vi "track2behavior.vi"(7 "ParallelPoolID":i32, 8 "error in (no error)":errorcluster, 10 "Track In":T2={"Track Centroid Positions (Camera Pixel)"=[], "Within Track Index"=0, "Camera Buffer Indecies"=[], "Area (Camera Pixels)"=0, "Speed (mm/s)"=0.0, "Direction (radians)"=0.0, "Centerline Positions (Camera Pixel)"=[], "Ellipse Ratio"=0.0, "Termination Reason"=enum."StillActive", "Track Index"=0, "Bounding Rect Left"=0, "Bounding Rect Top"=0, "Bounding Rect Right"=0, "Bounding Rect Bottom"=0, "Mature Camera Buffer"=-1, "Start Camera Buffer Index"=0, "Reverse Started Camera Buffer"=-1}, 11 "Original Worm Image":T1) -> (0 "error out":errorcluster, 2 "Track Out":T2={"Track Centroid Positions (Camera Pixel)"=[], "Within Track Index"=0, "Camera Buffer Indecies"=[], "Area (Camera Pixels)"=0, "Speed (mm/s)"=0.0, "Direction (radians)"=0.0, "Centerline Positions (Camera Pixel)"=[], "Ellipse Ratio"=0.0, "Termination Reason"=enum."StillActive", "Track Index"=0, "Bounding Rect Left"=0, "Bounding Rect Top"=0, "Bounding Rect Right"=0, "Bounding Rect Bottom"=0, "Mature Camera Buffer"=-1, "Start Camera Buffer Index"=0, "Reverse Started Camera Buffer"=-1})   [LabVIEW 2019]
uses:
  WormTrackSnippetCluster.ctl
  TrackTerminationReasonEnum.ctl
  <vilib>/vision/Image Controls.llb/IMAQ Image.ctl
  iterative_thinned_image_to_segment.vi
  pixel_XY_to_1D_index.vi
  thinned_image_to_centerline.vi/a49f2ef7-d53c-4424-bee3-5857753b5dab.vi
  iterative_segments_to_centerline.vi
  1D_index_to_pixel_XY.vi
  interp_1d_nearest.vi
  euclidean_distance_double.vi
  flip_2D_single_array_td.vi
  linspace_double.vi
  iterative_segments_to_centerline_oneiteration.vi
  DebugGlobal.vi
  ParametersGlobal.vi
  <vilib>/gmath/interp.llb/Search Ordered Table.vi
  <vilib>/vision/NI_Vision_Development_Module.lvlib
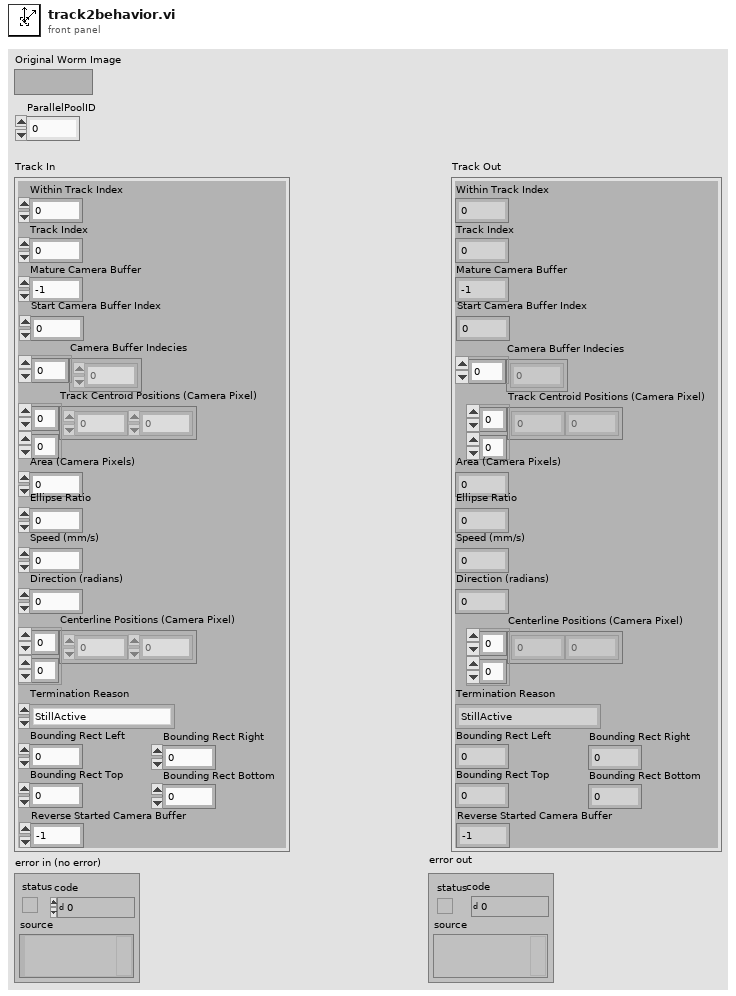
[diagram p1: front panel]
types:
  T1 = typedef "IMAQ Image.ctl" = refnum<image>
  T2 = typedef "WormTrackSnippetCluster.ctl" = cluster{"Track Centroid Positions (Camera Pixel)":sgl[][], "Within Track Index":i32, "Camera Buffer Indecies":i32[], "Area (Camera Pixels)":i32, "Speed (mm/s)":sgl, "Direction (radians)":sgl, "Centerline Positions (Camera Pixel)":sgl[][], "Ellipse Ratio":sgl, "Termination Reason":T3, "Track Index":i32, "Bounding Rect Left":i32, "Bounding Rect Top":i32, "Bounding Rect Right":i32, "Bounding Rect Bottom":i32, "Mature Camera Buffer":i32, "Start Camera Buffer Index":i32, "Reverse Started Camera Buffer":i32}
  T3 = typedef "TrackTerminationReasonEnum.ctl" = enum16{"StillActive", "MaxDisplacement", "NoBlobsLeft", "AreaIncrease", "AreaDecrease", "ExperimentEnded"}
  T4 = typedef "Particle Parameters" = i32
  T5 = cluster{"Left":i32, "Top":i32, "Right":i32, "Bottom":i32}
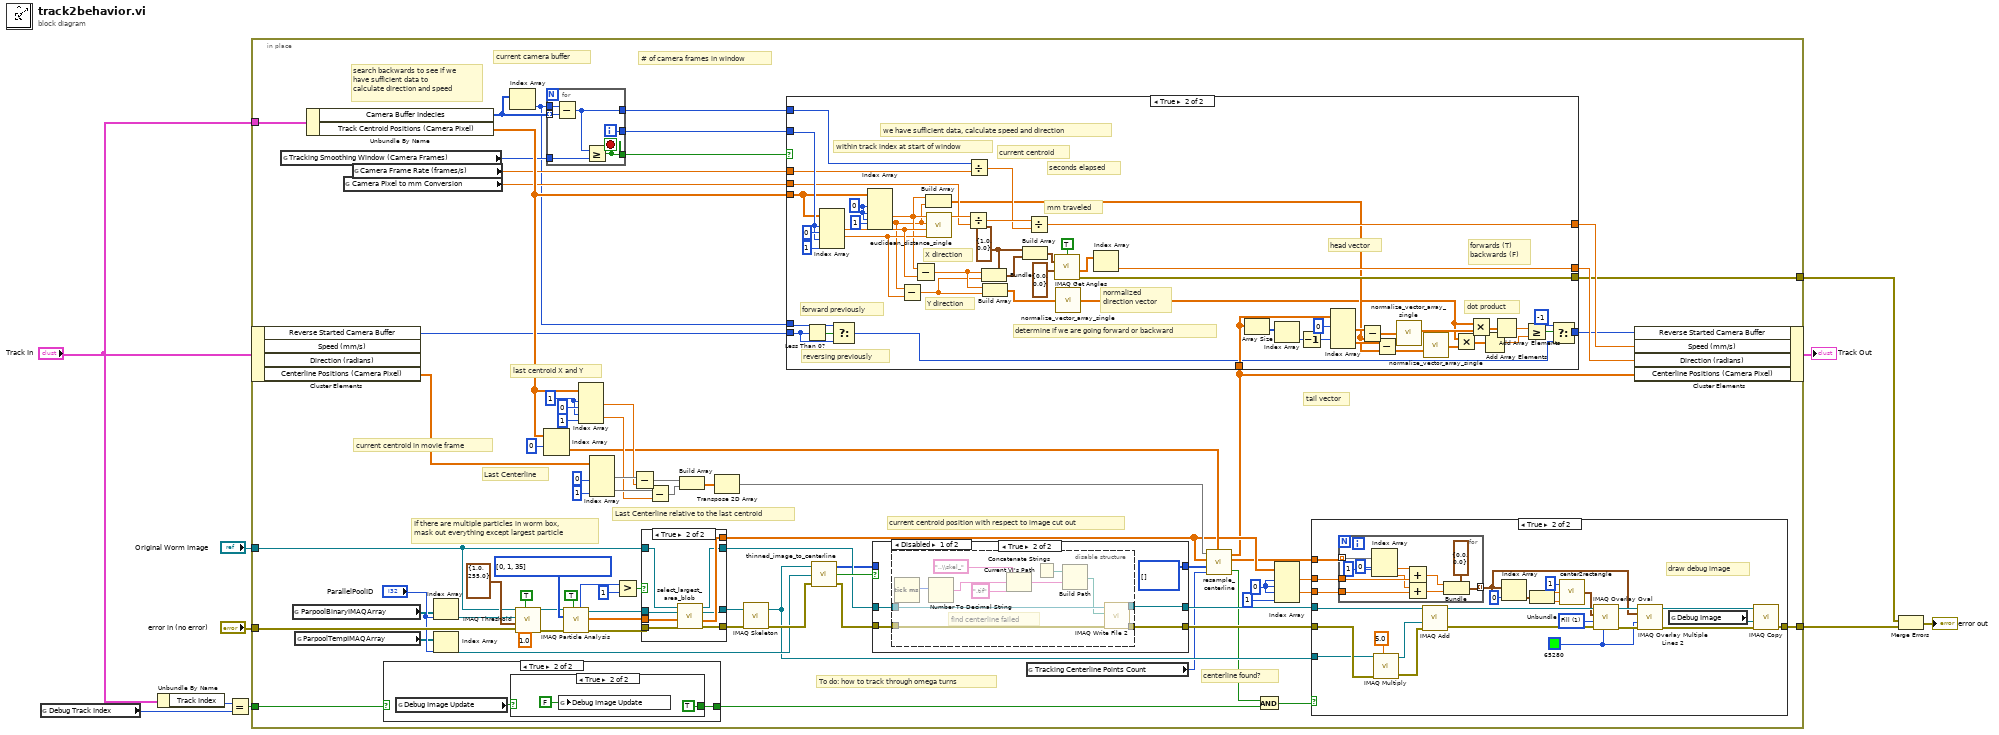
[diagram p0: block diagram]
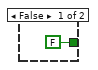
[diagram p2: hidden frame]
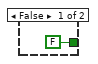
[diagram p3: hidden frame]
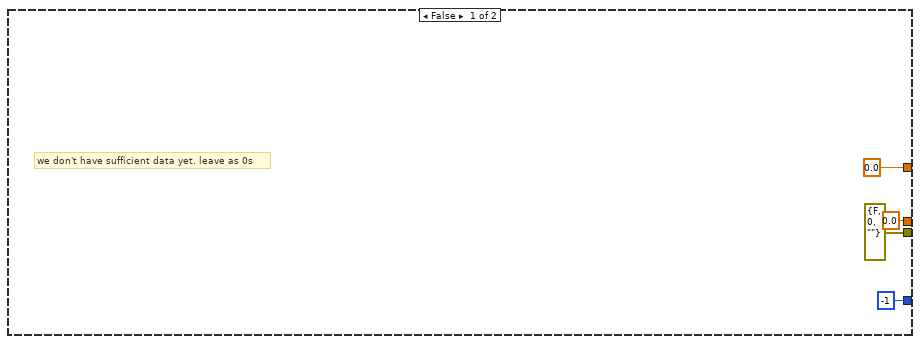
[diagram p8: hidden frame]
diagram:
  n1 = global read "DebugGlobal.vi" "Debug Track Index"() -> (w3:i32)
  n2 = Unbundle By Name("Track In") -> ("Track Index"=w4:i32)
  n3 = Equal?(x=w4, y=w3) -> (x = y?=w2:bool)
  n4 = in-place {
    in-place-border: "Track In" -> [w27]
    in-place-border: "error in (no error)" -> [w79]
    in-place-border: [w25] -> w7
    in-place-border: "Original Worm Image" -> [w65]
    in-place-border: [w66] -> w5
    in-place-border: w2 -> [w12]
    w22 = 1 ("index (row)")
    w36 = 0 ("index (row)")
    w75 = T4[] [0, 1, 35] items=["Center of Mass X", "Center of Mass Y", "First Pixel X", "First Pixel Y", "Bounding Rect Left", "Bounding Rect Top", "Bounding Rect Right", "Bounding Rect Bottom", "Max Feret Diameter Start X", "Max Feret Diameter Start Y", "Max Feret Diameter End X", "Max Feret Diameter End Y", "Max Horiz. Segment Length Left", "Max Horiz. Segment Length Right", "Max Horiz. Segment Length Row", "-", "Bounding Rect Width", "Bounding Rect Height", "Bounding Rect Diagonal", "Perimeter", "Convex Hull Perimeter", "Holes' Perimeter", "Max Feret Diameter", "Equivalent Ellipse Major Axis", "Equivalent Ellipse Minor Axis", "Equivalent Ellipse Minor Axis (Feret)", "Equivalent Rect Long Side", "Equivalent Rect Short Side", "Equivalent Rect Diagonal", "Equivalent Rect Short Side (Feret)", "Average Horiz. Segment Length", "Average Vert. Segment Length", "Hydraulic Radius", "Waddel Disk Diameter", "-", "Area", "Holes' Area", "Particle & Holes' Area", "Convex Hull Area", "Image Area", "-", "Number of Holes", "Number of Horiz. Segments", "Number of Vert. Segments", "-", "Orientation", "Max Feret Diameter Orientation", "-", "% Area/Image Area", "% Area/(Particle & Holes' Area)", "Ratio of Equivalent Ellipse Axes", "Ratio of Equivalent Rect Sides", "-", "Elongation Factor", "Compactness Factor", "Heywood Circularity Factor", "Type Factor", "-", "Sum X", "Sum Y", "Sum XX", "Sum XY", "Sum YY", "Sum XXX", "Sum XXY", "Sum XYY", "Sum YYY", "-", "Moment of Inertia XX", "Moment of Inertia XY", "Moment of Inertia YY", "Moment of Inertia XXX", "Moment of Inertia XXY", "Moment of Inertia XYY", "Moment of Inertia YYY", "Norm. Moment of Inertia XX", "Norm. Moment of Inertia XY", "Norm. Moment of Inertia YY", "Norm. Moment of Inertia XXX", "Norm. Moment of Inertia XXY", "Norm. Moment of Inertia XYY", "Norm. Moment of Inertia YYY", "Hu Moment 1", "Hu Moment 2", "Hu Moment 3", "Hu Moment 4", "Hu Moment 5", "Hu Moment 6", "Hu Moment 7"] ("Pixel Measurements")
    # "current camera buffer"
    # "tail vector"
    # "# of camera frames in window"
    # "If there are multiple particles in worm box, \nmask out everything except largest particle"
    # "centerline found?"
    # "current centroid position with respect to image cut out"
    # "To do: how to track through omega turns"
    # "current centroid in movie frame"
    # "Last Centerline"
    # "last centroid X and Y"
    # "Last Centerline relative to the last centroid"
    # "search backwards to see if we \nhave sufficient data to \ncalculate direction and speed"
    n5 = in-place-cluster #1("Track In") -> ("Reverse Started Camera Buffer"=w18:i32, "Centerline Positions (Camera Pixel)"=w54:sgl[][])  [unwired: 2 out]
    n6 = global read "ParametersGlobal.vi" "Tracking Smoothing Window (Camera Frames)"() -> (w32:i32)
    n7 = global read "ParametersGlobal.vi" "ParpoolBinaryIMAQArray"() -> (w28:T1[])
    n8 = global read "ParametersGlobal.vi" "ParpoolTempIMAQArray"() -> (w29:T1[])
    n9 = Unbundle By Name(w27) -> ("Camera Buffer Indecies"=w84:i32[], "Track Centroid Positions (Camera Pixel)"=w41:sgl[][])
    n10 = global read "ParametersGlobal.vi" "Camera Pixel to mm Conversion"() -> (w30:sgl)
    n11 = global read "ParametersGlobal.vi" "Camera Frame Rate (frames/s)"() -> (w31:sgl)
    n12 = case shown="True" w12 {
      tunnel: [FALSE w87] -> w11
      frame False {
      }
      frame True {
        n13 = global read "DebugGlobal.vi" "Debug Image Update"() -> (w88:bool)
        n14 = case shown="True" w88 {
          tunnel: [FALSE TRUE] -> w87
          frame False {
          }
          frame True {
            n15 = global write "DebugGlobal.vi" "Debug Image Update"(FALSE ("Debug Image Update")) -> ()
          }
        }
      }
    }
    n16 = Index Array(array=w28, index="ParallelPoolID") -> (element=w26:T1)
    n17 = Index Array(array=w29, index="ParallelPoolID") -> (element=w62:T1)
    n18 = Index Array(array=w84) -> (element=w13:i32)  [unwired: 1 in]
    n19 = call "IMAQ Threshold"("Replace Value"=sgl 1.0, "Keep/Replace Value (Replace)"=TRUE, "error in (no error)"=w79, "Range"=cluster{"Lower value":sgl, "Upper value":sgl} {"Lower value"=1.0, "Upper value"=255.0}, "Image Dst"=w26, "Image Src"=w65) -> ("error out"=w77:errorcluster, "Image Dst Out"=w64:T1)  [unwired: 4 in]
    n20 = Index Array(array=w41, index (row)=0) -> (element=w39:sgl[])  [unwired: 1 in]
    n21 = for {
      tunnel: w84 -> [w163] mode=indexing
      tunnel: w13 -> [w168]
      tunnel: [w164] -> w82
      tunnel: w32 -> [w167]
      tunnel: [w166] -> w83
      tunnel: [w165] -> w43
      i -> [w164]
      stop <- w166 stop-if-true
      n22 = Subtract(x=w168, y=w163) -> (x-y=w165:i32)
      n23 = Greater Or Equal?(x=w165, y=w167) -> (x >= y?=w166:bool)
    }
    n24 = call "IMAQ Particle Analysis"("Connectivity 4/8 (8)"=TRUE, "error in (no error)"=w77, "Pixel Measurements"=w75, "Image"=w64) -> ("error out"=w74:errorcluster, "Particle Measurements (Pixels)"=w72:dbl[][], "Image Out (duplicate)"=w73:T1, "Number of Particles"=w76:i32)  [unwired: 2 in, 2 out]
    n25 = Index Array(array=w41, index (row) #1=w22, index (col) #1=0 ("disabled index (col)"), index (row) #2=w22, index (col) #2=1 ("index (col)")) -> (element #1=w52:sgl, element #2=w50:sgl)
    n26 = Index Array(array=w54, index (col) #1=0 ("disabled index (col)"), index (col) #2=1 ("index (col)")) -> (element #1=w53:sgl[], element #2=w51:sgl[])  [unwired: 2 in]
    n27 = Greater?(x=w76, y=1) -> (0:w80:bool)
    n28 = Subtract(x=w53, y=w52) -> (x-y=w49:sgl[])
    n29 = case shown="True" w80 {
      tunnel: w73 -> [w152 w161]
      tunnel: w74 -> [w153 w162]
      tunnel: w65 -> [w154 w159]
      tunnel: [w154 w156] -> w58
      tunnel: [w153 w158] -> w19
      tunnel: [w152 w155] -> w20
      tunnel: w72 -> [w151 w160]
      tunnel: [w151 w157] -> w33
      frame False {
      }
      frame True {
        n30 = call "select_largest_area_blob.vi"("error in (no error)"=w162, "Particle Measurements (Pixels) In"=w160, "Binary Image In"=w161, "Original Image In"=w159) -> ("error out"=w158:errorcluster, "Particle Measurements (Pixels) Out"=w157:dbl[][], "Binary Image Out"=w155:T1, "Original Image Out"=w156:T1)
      }
    }
    n31 = Subtract(x=w51, y=w50) -> (x-y=w48:sgl[])
    n32 = Build Array(w49, w48) -> (w47:sgl[][])
    n33 = Transpose 2D Array(2D array=w47) -> (transposed array=w40:sgl[][])
    n34 = call "IMAQ Skeleton"("error in (no error)"=w19, "Image Src"=w20) -> ("error out"=w63:errorcluster, "Image Dst Out"=w61:T1)  [unwired: 4 in]
    n35 = call "thinned_image_to_centerline.vi"("error in"=w63, "Temp Image"=w62, "Skeleton Image"=w61) -> ("error out"=w56:errorcluster, "Algorithm timed out"=w59:bool, "Centline Pixels"=w57:i32[][])
    n36 = case shown="True" w59 {
      tunnel: w58 -> [w92 w99]
      tunnel: w57 -> [w94 _]
      tunnel: [w94 i32[][] [] ("tip pixels")] -> w46
      tunnel: w56 -> [w93 w97]
      tunnel: [w93 w96] -> w55
      tunnel: [w92 w95] -> w44
      frame False {
      }
      frame True {
        n37 = disable-structure shown="Disabled" {
          disable-tunnel: w99 -> [w110 w112]
          disable-tunnel: w97 -> [w106 w111]
          disable-tunnel: [w105 w111] -> w96
          disable-tunnel: [w104 w112] -> w95
          frame Disabled {
            # "find centerline failed"
            n38 = Tick Count (ms)() -> (millisecond timer value=w109:u32)
            n39 = Number To Decimal String(number=w109) -> (decimal integer string=w108:string)  [unwired: 1 in]
            n40 = Concatenate Strings("..\\skel_", w108, ".tif" ("string")) -> (w101:string)
            n41 = Current VI's Path() -> (path=w100:path)
            n42 = Build Path(base path=w100, name or relative path=w101) -> (appended path=w102:path)
            n43 = call-poly "IMAQ Write File 2"("error in (no error)"=w106, "File Path"=w102, "Image"=w110) -> ("error out"=w105:errorcluster, "Image Out (duplicate)"=w104:T1)  [unwired: 7 in]
          }
          frame Enabled {
          }
        }
      }
    }
    n44 = global read "ParametersGlobal.vi" "Tracking Centerline Points Count"() -> (w16:i32)
    n45 = call "resample_centerline.vi"("Last Centerline (last centroid)"=w40, "Centroid (bounding rectangle)"=w33, "Centerline Pixels"=w46, "Sample Points"=w16, "current centroid (camera origin)"=w39) -> ("Centerline (camera origin)"=w15:sgl[][], "Centerline (bounding rectangle)"=w17:sgl[][], "Centerline found?"=w38:bool)
    n46 = case shown="True" w83 {
      tunnel: [sgl 0.0 w207] -> w85
      tunnel: [sgl 0.0 ("Angle (deg)") w206] -> w42
      tunnel: w31 -> [_ w210]
      tunnel: w82 -> [_ w221]
      tunnel: w41 -> [_ w220]
      tunnel: w30 -> [_ w209]
      tunnel: [errorcluster {"status"=FALSE, "code"=0, "source"=""} ("error out") w212] -> w25
      tunnel: w43 -> [_ w211]
      tunnel: w18 -> [_ w176]
      tunnel: w15 -> [_ w183]
      tunnel: [-1 ("Reverse Started Camera Buffer") w179] -> w14
      tunnel: w13 -> [_ w177]
      frame False {
        # "we don't have sufficient data yet. leave as 0s"
      }
      frame True {
        w197 = cluster{"X":sgl, "Y":sgl} {"X"=1.0, "Y"=0.0} ("Vertex")
        w208 = 0 ("disabled index (col)")
        # "determine if we are going forward or backward"
        # "forward previously"
        # "reversing previously"
        # "forwards (T)\nbackwards (F)"
        # "dot product"
        # "current centroid"
        # "normalized\ndirection vector"
        # "head vector"
        # "Y direction"
        # "X direction"
        # "within track index at start of window"
        # "mm traveled"
        # "seconds elapsed"
        # "we have sufficient data, calculate speed and direction"
        n47 = Less Than 0?(x=w176) -> (x < 0?=w178:bool)
        n48 = Index Array(array=w220, index (row) #1=w221, index (col) #1=0 ("disabled index (col)"), index (row) #2=w221, index (col) #2=1 ("index (col)")) -> (element #1=w205:sgl, element #2=w204:sgl)
        n49 = Select(t=w177, s=w178, f=w176) -> (s? t:f=w175:i32)
        n50 = Index Array(array=w220, index (row) #1=w208, index (col) #1=w208, index (row) #2=w208, index (col) #2=1 ("index (col)")) -> (element #1=w196:sgl, element #2=w195:sgl)
        n51 = Subtract(x=w195, y=w204) -> (x-y=w201:sgl)
        n52 = Subtract(x=w196, y=w205) -> (x-y=w202:sgl)
        n53 = Build Array(w196, w195) -> (w192:sgl[])
        n54 = call "euclidean_distance_single.vi"("Point 2 Y"=w204, "Point 2 X"=w205, "Point 1 Y"=w195, "Point 1 X"=w196) -> ("Distance"=w219:sgl)  [unwired: 7 in]
        n55 = Divide(x=w219, y=w209) -> (x/y=w218:sgl)
        n56 = Divide(x=w211, y=w210) -> (x/y=w217:sgl)
        n57 = Bundle(cluster=w197, "X"=w202, "Y"=w201) -> (w203:cluster{"X":sgl, "Y":sgl})
        n58 = Build Array(w202, w201) -> (w200:sgl[])
        n59 = Build Array(w197, w203) -> (w214:cluster{"X":sgl, "Y":sgl}[])
        n60 = Divide(x=w218, y=w217) -> (x/y=w207:sgl)
        n61 = call "IMAQ Get Angles"("Vertex"=cluster{"X":sgl, "Y":sgl} {"X"=0.0, "Y"=0.0}, "Points"=w214, "Use Vertex (No)"=TRUE) -> ("error out"=w212:errorcluster, "Angles (rad)"=w213:sgl[])  [unwired: 2 in, 1 out]
        n62 = call "normalize_vector_array_single.vi"("2 element vector"=w200) -> ("normalized vector out"=w187:sgl[])
        n63 = Index Array(array=w213) -> (element=w206:sgl)  [unwired: 1 in]
        n64 = Array Size(array=w183) -> (size(s)=w184:i32[])
        n65 = Index Array(array=w184) -> (element=w182:i32)  [unwired: 1 in]
        n66 = Decrement(x=w182) -> (x-1=w199:i32)
        n67 = Index Array(array=w183, index (row) #1=0 ("index (row)"), index (row) #2=w199) -> (element #1=w194:sgl[], element #2=w193:sgl[])  [unwired: 2 in]
        n68 = Subtract(x=w194, y=w192) -> (x-y=w190:sgl[])
        n69 = Subtract(x=w193, y=w192) -> (x-y=w191:sgl[])
        n70 = call "normalize_vector_array_single.vi"("2 element vector"=w190) -> ("normalized vector out"=w189:sgl[])
        n71 = call "normalize_vector_array_single.vi"("2 element vector"=w191) -> ("normalized vector out"=w188:sgl[])
        n72 = Multiply(x=w187, y=w188) -> (x*y=w185:sgl[])
        n73 = Multiply(x=w187, y=w189) -> (x*y=w186:sgl[])
        n74 = Add Array Elements(numeric array=w185) -> (sum=w173:sgl)
        n75 = Add Array Elements(numeric array=w186) -> (sum=w174:sgl)
        n76 = Greater Or Equal?(x=w174, y=w173) -> (x >= y?=w181:bool)
        n77 = Select(t=-1 ("Reverse Started Camera Buffer"), s=w181, f=w175) -> (s? t:f=w179:i32)
      }
    }
    n78 = And(x=w38, y=w11) -> (x .and. y?=w45:bool)
    n79 = Index Array(array=w33, index (row) #1=w36, index (col) #1=w36, index (row) #2=w36, index (col) #2=1 ("disabled index (col)")) -> (element #1=w35:dbl, element #2=w34:dbl)
    n80 = case shown="True" w45 {
      tunnel: w55 -> [w113 w139]
      tunnel: w44 -> [_ w134]
      tunnel: [w113 w132] -> w66
      tunnel: w61 -> [_ w136]
      tunnel: w17 -> [_ w129]
      tunnel: w35 -> [_ w128]
      tunnel: w34 -> [_ w127]
      frame False {
      }
      frame True {
        w123 = u32 1 items=["Frame", "Fill"] ("Drawing Mode (Frame)")
        w124 = u32 65280 ("Color")
        # "draw debug image"
        n81 = for {
          tunnel: [w147] -> w119 mode=indexing
          tunnel: w129 -> [w146] mode=indexing
          tunnel: w128 -> [w144]
          tunnel: w127 -> [w141]
          n82 = Index Array(array=w146, index #1=0 ("index"), index #2=1 ("index")) -> (element #1=w145:sgl, element #2=w142:sgl)
          n83 = Add(x=w145, y=w144) -> (x+y=w143:dbl)
          n84 = Add(x=w142, y=w141) -> (x+y=w140:dbl)
          n85 = Bundle(cluster=cluster{"X":dbl, "Y":dbl} {"X"=0.0, "Y"=0.0} ("Point Coordinates"), "X"=w143, "Y"=w140) -> (w147:cluster{"X":dbl, "Y":dbl})
        }
        n86 = call "IMAQ Multiply"("Image Src A"=w136, "Constant"=5.0, "error in (no error)"=w139) -> ("Image Dst Out"=w135:T1, "error out"=w137:errorcluster)  [unwired: 4 in]
        n87 = call "IMAQ Add"("Image Src A"=w134, "Image Src B"=w135, "error in (no error)"=w137) -> ("Image Dst Out"=w122:T1, "error out"=w126:errorcluster)  [unwired: 4 in]
        n88 = Index Array(array=w119, index=0) -> (element=w117:cluster{"X":dbl, "Y":dbl})
        n89 = Unbundle(w117) -> ("X"=w116:dbl, "Y"=w115:dbl)
        n90 = call "center2rectangle.vi"("Center Y"=w115, "Center X"=w116, "Box Half Size"=1) -> ("Box Rectangle"=w114:T5)
        n91 = call "IMAQ Overlay Oval"("Color"=w124, "error in (no error)"=w126, "Drawing Mode (Frame)"=w123, "Bounding Rectangle"=w114, "Image"=w122) -> ("error out"=w125:errorcluster, "Image Out"=w121:T1)  [unwired: 5 in]
        n92 = call "IMAQ Overlay Multiple Lines 2"("Image"=w121, "Line End Points"=w119, "Color"=w124, "error in (no error)"=w125) -> ("Image Out"=w130:T1, "error out"=w133:errorcluster)  [unwired: 10 in]
        n93 = global read "DebugGlobal.vi" "Debug Image"() -> (w131:T1)
        n94 = call "IMAQ Copy"("error in (no error)"=w133, "Image Dst"=w131, "Image Src"=w130) -> ("error out"=w132:errorcluster)  [unwired: 3 in, 1 out]
      }
    }
    n95 = in-place-cluster #1("Reverse Started Camera Buffer"=w14, "Speed (mm/s)"=w85, "Direction (radians)"=w42, "Centerline Positions (Camera Pixel)"=w15) -> (→"Track Out":T2)
  }
  n96 = Merge Errors(w7, w5) -> (→"error out":errorcluster)
